vi "Build IPK.vi"(5 "Files Generated by Build":path[](array[path]), 6 "Top Level/Always Included VIs":path[](array[path]), 7 "Destination Path":path, 8 "error in (no error)":errorcluster, 9 "Target Name":string, 10 "Build Specification Name":string, 11 "Project Path":path) -> (0 "error out":errorcluster)   [LabVIEW 2015]
panel:
  out "command line":string
  out "standard error":string
  out "standard output":string
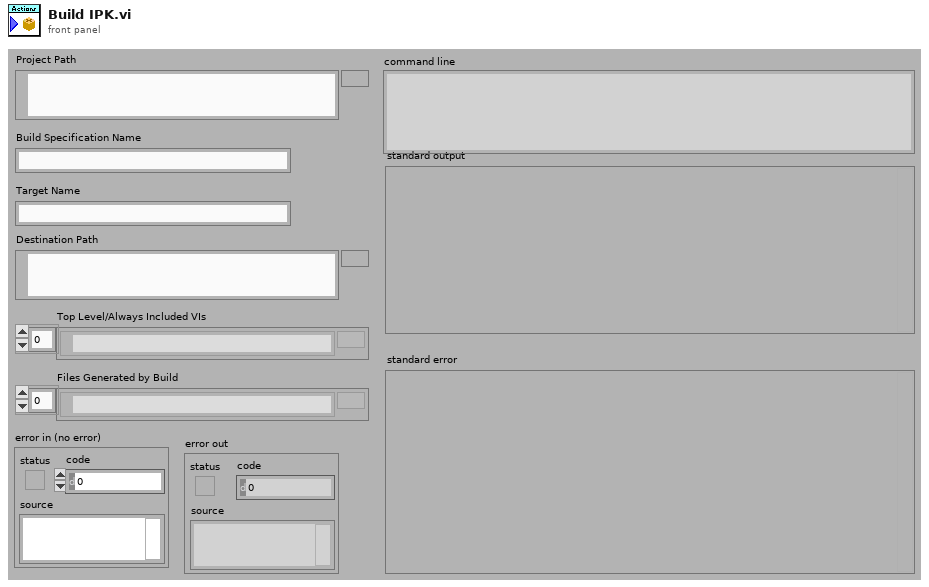
[diagram p1: front panel]
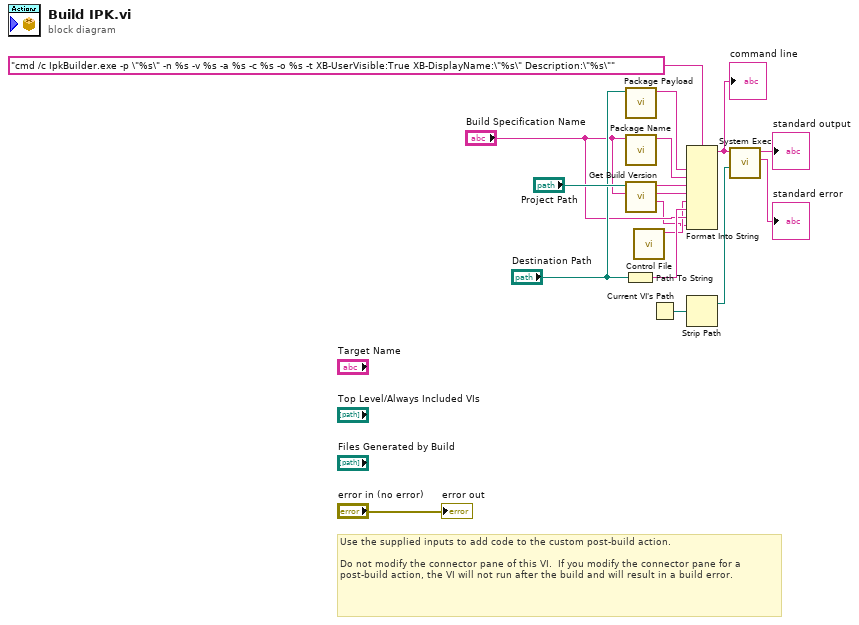
[diagram p0: block diagram]
diagram:
  # "Use the supplied inputs to add code to the custom post-build action.\n\nDo not modify the connector pane of this VI.  If you modify the connector pane for a post-build action, the VI will not run after the build and will result in a build error."
  n1 = Path To String(path="Destination Path") -> (string=w5:string)
  n2 = call "Package Payload.vi"("Destination Path"="Destination Path") -> ("String"=w8:string)  [unwired: 10 in]
  n3 = call "Package Name.vi"("Build Specification Name"="Build Specification Name") -> ("Package Name"=w9:string)  [unwired: 10 in]
  n4 = call "Get Build Version.vi"("Build Spec Name"="Build Specification Name", "Project Path"="Project Path") -> ("Description"=w1:string, "Architecture"=w6:string, "Package Version"=w7:string)  [unwired: 6 in, 1 out]
  n5 = call "Control File.vi"() -> ("Control File"=w2:string)  [unwired: 11 in]
  n6 = Current VI's Path() -> (path=w13:path)
  n7 = Format Into String(format string="cmd /c IpkBuilder.exe -p \"%s\" -n %s -v %s -a %s -c %s -o %s -t XB-UserVisible:True XB-DisplayName:\"%s\" Description:\"%s\"", w8, w9, w7, w6, w2, w5, "Build Specification Name", w1) -> (resulting string=w10:string)  [unwired: 2 in, 1 out]
  "command line" <- w10
  n8 = Strip Path(path=w13) -> (stripped path=w12:path)  [unwired: 1 out]
  n9 = call <vilib>:"System Exec.vi"("working directory"=w12, "command line"=w10) -> ("standard error"=→"standard error":string, "standard output"=→"standard output":string)  [unwired: 6 in, 2 out]
  "error out" <- "error in (no error)"
